vi "Read Selected Tests.vi"(8 "error in (no error)":errorcluster, 11 "Test Selector in":refnum<class "Test Selector.lvclass">) -> (0 "error out":errorcluster, 2 "Selected Tests":bool[](array[boolean]), 3 "Test Selector out":refnum<class "Test Selector.lvclass">)   [LabVIEW 2019, in "Test Selector.lvlib" / "Test Selector.lvclass"]
uses:
  Test Selector.lvclass
  Test Selector.lvclass/Test Selector.ctl
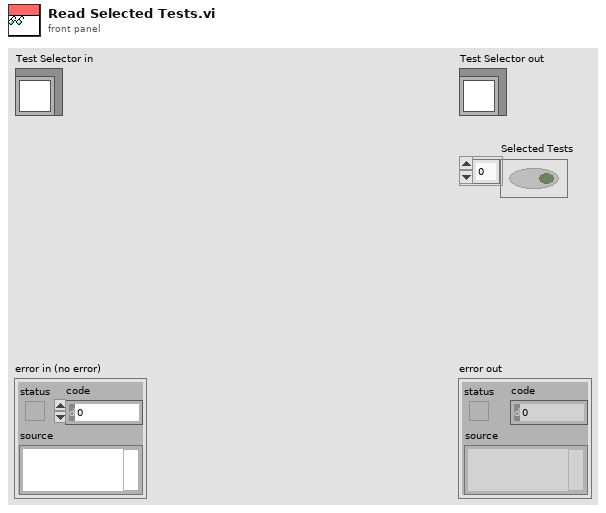
[diagram p1: front panel]
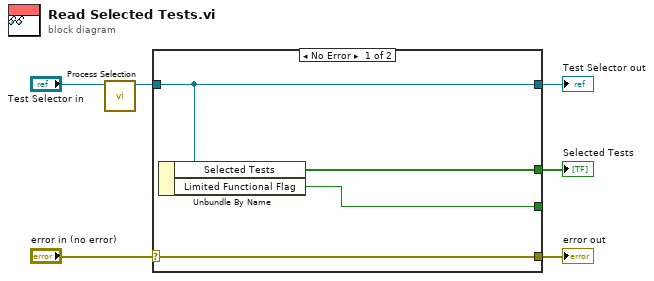
[diagram p0: block diagram]
diagram:
  n1 = call "Process Selection.vi"("Test Selector in"="Test Selector in") -> ("Test Selector out"=w1:refnum<class "Test Selector.lvclass">)  [unwired: 9 in, 1 out]
  n2 = case shown="No Error" "error in (no error)" {
    selector: "error in (no error)" -> [w10 w11]
    tunnel: [w10 w11] -> w5
    tunnel: [w9 w12] -> w4
    tunnel: w1 -> [w9 w12]
    tunnel: [w8 _] -> w3
    tunnel: [w7 _] -> _
    frame No Error {
      n3 = Unbundle By Name(w9) -> ("Selected Tests"=w8:bool[], "Limited Functional Flag"=w7:bool)
    }
    frame Error {
    }
  }
  "error out" <- w5
  "Test Selector out" <- w4
  "Selected Tests" <- w3
